vi "Get Array of Record Data.vi"(8 "error in (no error)":errorcluster, 11 "Record.Error in":refnum<class "Record.Error.lvclass">) -> (0 "error out":errorcluster, 2 "Array of Record Data":variant[](array[variant]), 3 "Record.Error out":refnum<class "Record.Error.lvclass">)   [LabVIEW 2017, in "Error Log.lvlib" / "Record.Error.lvclass"]
uses:
  Record.Error.lvclass
  Record.Error.lvclass/Record.Error.ctl
  Record/Record.lvclass
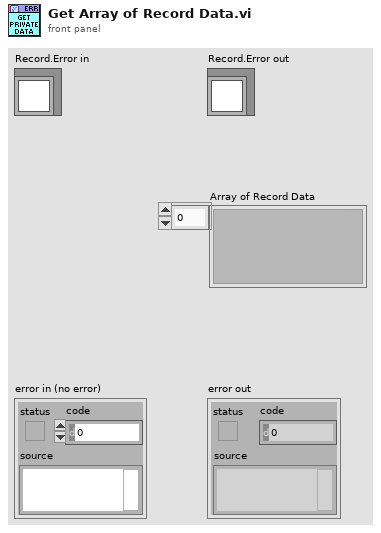
[diagram p1: front panel]
types:
  T1 = typedef "Error Log.lvlib/Record.Error.lvclass/Private Data.ctl" = cluster{"Call Chain":string, "Error":errorcluster}
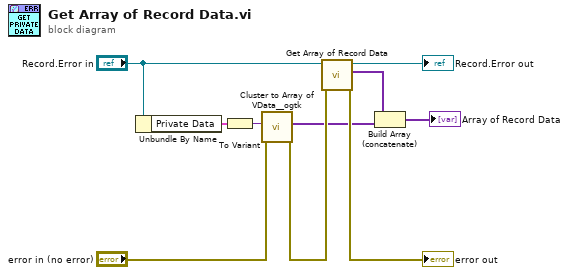
[diagram p0: block diagram]
diagram:
  n1 = Unbundle By Name("Record.Error in") -> ("Private Data"=w10:T1)
  n2 = To Variant(anything=w10) -> (Variant=w7:variant)
  n3 = call <userlib>:"Cluster to Array of VData__ogtk.vi"("error in (no error)"="error in (no error)", "Cluster"=w7) -> ("error out"=w3:errorcluster, "Array of VData"=w1:variant[])  [unwired: 8 in]
  n4 = call-parent "Get Array of Record Data.vi"("error in (no error)"=w3, "Record in"="Record.Error in") -> ("error out"=→"error out":errorcluster, "Array of Record Data"=w5:variant[], "Record out"=→"Record.Error out":refnum<class "Record.Error.lvclass">)  [unwired: 7 in]
  n5 = Build Array (concatenate)(w5, w1) -> (→"Array of Record Data":variant[])
